vi "Cooler Panel UI Components.vi"() -> ()   [LabVIEW 2012]
doc: "This is Actor Core.vi, the main message handling loop for Actors. An actor usually just sits in this loop and processes messages as they arrive. Any error returned by the message Do.vi call will stop the loop, with error code 43 as the cannonical signal to stop with no error sent to caller. Descendants may override that in Handle Error.vi."
panel:
  out "Pump":bool
  out "Fault B":bool
  in  "Desired Temperature":dbl=75.0
  out "Temperature":dbl(slide) scale=0.0..120.0
  out "Fault A":bool
  out "Fan B":bool
  out "Fan A":bool
  # "Fan starts 5 seconds after pump starts"
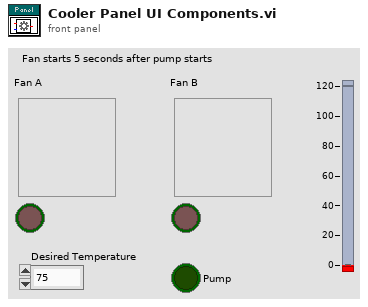
[diagram p1: front panel]
types:
  T1 = enum32{"Invalid", "Standard", "Closed", "Hidden", "Minimized", "Maximized"}
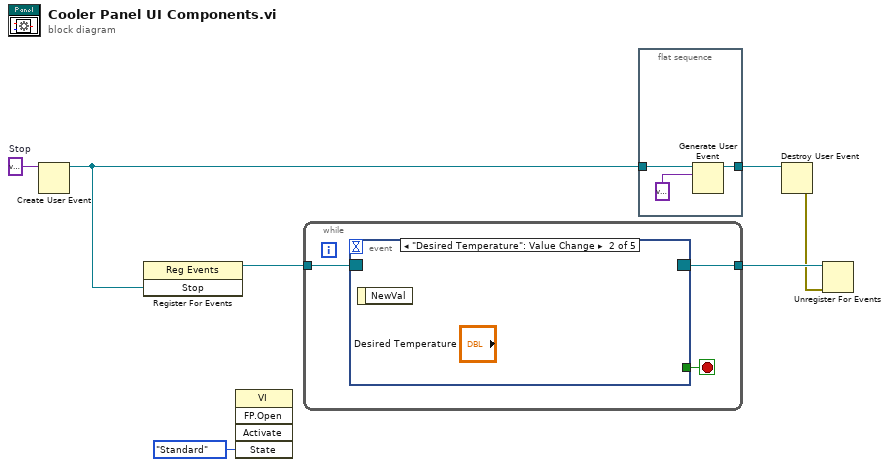
[diagram p0: block diagram]
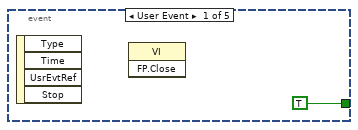
[diagram p2: hidden frame]
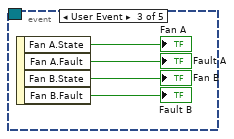
[diagram p3: hidden frame]
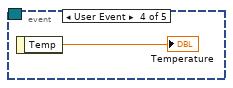
[diagram p4: hidden frame]
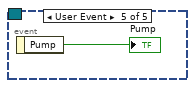
[diagram p5: hidden frame]
diagram:
  w6 = variant  # Stop
  n1 = Create User Event(user event datatype=w6) -> (user event=w1:refnum<user-event>)  [unwired: 1 in, 1 out]
  n2 = register-events(w1) -> (reference out=w7:refnum<event-registration>)  [unwired: 2 in, 1 out]
  n3 = invoke class="VI" method="FP.Open"("State"=T1."Standard") -> ()  [unwired: 4 in, 5 out]
  n4 = while {
    tunnel: w7 -> [w10]
    tunnel: [w9] -> w5
    stop <- w8 stop-if-true
    n5 = event shown="[1] \"Desired Temperature\": Value Change" {
      selector: w10 -> [_ _ _ _ _]
      dyn-events: [_ _ _ _ _] -> w9
      timeout: _ -> [_ _ _ _ _]
      tunnel: [TRUE _ _ _ _] -> w8
      event User Event {
        n6 = event-data() -> ()  [unwired: 1 in, 4 out]
        n7 = invoke class="VI" method="FP.Close"() -> ()  [unwired: 3 in, 3 out]
      }
      event "Desired Temperature": Value Change {
        n8 = event-data() -> ()  [unwired: 1 in, 1 out]
      }
      event User Event {
        n9 = event-data() -> ("Fan A.State"=→"Fan A":bool, "Fan A.Fault"=→"Fault A":bool, "Fan B.State"=→"Fan B":bool, "Fan B.Fault"=→"Fault B":bool)  [unwired: 1 in]
      }
      event User Event {
        n10 = event-data() -> ("Temp"=→"Temperature":dbl)  [unwired: 1 in]
      }
      event User Event {
        n11 = event-data() -> ("Pump"=→"Pump":bool)  [unwired: 1 in]
      }
    }
  }
  n12 = flat-sequence {
    tunnel: [w20] -> w3
    tunnel: w1 -> [w19]
    frame #0 {
      n13 = Generate User Event(user event=w19, event data cluster=variant ("Stop")) -> (user event out=w20:refnum<user-event>)  [unwired: 1 in, 1 out]
    }
  }
  n14 = Destroy User Event(user event=w3) -> (error out=w4:errorcluster)  [unwired: 1 in]
  n15 = Unregister For Events(event registration refnum=w5, error in=w4) -> ()  [unwired: 1 out]
